vi "Update Settings.vi"(8 "error in (no error)":errorcluster, 10 "Settings":T1={"Port"="", "BaudRate"=9600, "Wakeup Signal Address "=0, "Acquisiton Address"=0, "Acknowledgement Address"=0, "Sleep Address"=0}, 11 "PLCHandler in":refnum<class "PLCHandler.lvclass">) -> (0 "error out":errorcluster, 3 "PLCHandler out":refnum<class "PLCHandler.lvclass">)   [LabVIEW 2022 SP3, in "PLCHandler.lvlib" / "PLCHandler.lvclass"]
uses:
  PLCHandler.lvclass
  PLCHandler.lvclass/PLCHandler.ctl
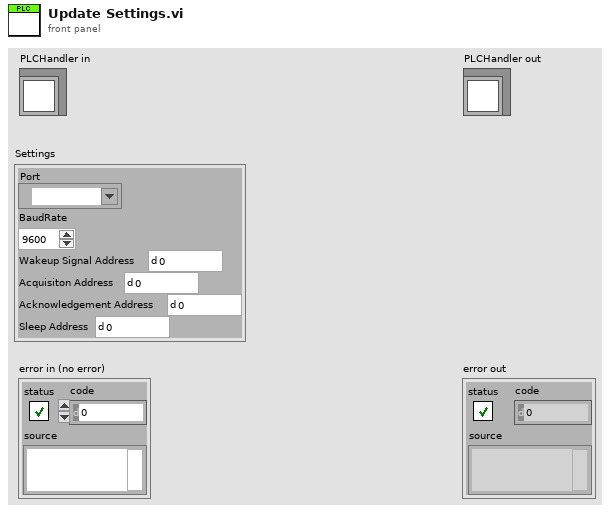
[diagram p1: front panel]
types:
  T1 = cluster{"Port":refnum<visa-resource-name>, "BaudRate":u32, "Wakeup Signal Address ":u16, "Acquisiton Address":u16, "Acknowledgement Address":u16, "Sleep Address":u16}
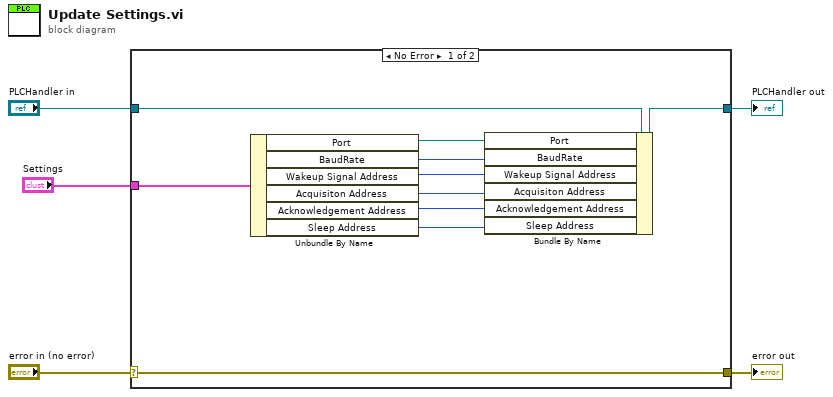
[diagram p0: block diagram]
diagram:
  n1 = case shown="No Error" "error in (no error)" {
    selector: "error in (no error)" -> [w14 w17]
    tunnel: [w14 w17] -> w4
    tunnel: [w13 w16] -> w2
    tunnel: "PLCHandler in" -> [w15 w16]
    tunnel: "Settings" -> [w12 _]
    frame No Error {
      n2 = Unbundle By Name(w12) -> ("Port"=w6:refnum<visa-resource-name>, "BaudRate"=w7:u32, "Wakeup Signal Address"=w8:u16, "Acquisiton Address"=w9:u16, "Acknowledgement Address"=w10:u16, "Sleep Address"=w11:u16)
      n3 = Bundle By Name(cluster=w15, "Port"=w6, "BaudRate"=w7, "Wakeup Signal Address"=w8, "Acquisiton Address"=w9, "Acknowledgement Address"=w10, "Sleep Address"=w11) -> (w13:refnum<class "PLCHandler.lvclass">)
    }
    frame Error {
    }
  }
  "error out" <- w4
  "PLCHandler out" <- w2
